vi "Test Get Sender from Nested Call Chain on Send.vi"(8 "error in (no error)":errorcluster, 11 "Test Case In":refnum<class "Debug Data Test.lvclass">) -> (0 "error out":errorcluster, 3 "Test Case Out":refnum<class "Debug Data Test.lvclass">)   [LabVIEW 2020, in "Debug Data Test.lvclass"]
uses:
  Debug Data Test.lvclass
  C:/Program Files (x86)/National Instruments/LabVIEW 2020/vi.lib/Astemes/LUnit/Test Case.lvclass
  source/Debug Data/Raw Debug Data.ctl
  source/Debug Data/Debug Data.lvclass/Debug Data.ctl
  <vilib>/Astemes/LUnit/Test Case.lvclass/Test Case.ctl
  <vilib>/Astemes/LUnit/LUnit Assertion Result.lvclass/LUnit Assertion Result.ctl
  <vilib>/Astemes/LUnit/LUnit Test Case Result.lvclass/LUnit Test Case Result.ctl
  <vilib>/Astemes/LUnit/LUnit Method Result.lvclass/LUnit Method Result.ctl
  01074fa8-ee8a-411d-bc8b-fc92c4f90959.vi
  <vilib>/Astemes/LUnit/Palette/Pass.vi
  <vilib>/Astemes/LUnit/Palette/Fail.vi
  <vilib>/Astemes/LUnit/Compare Variants.vi
  <vilib>/Astemes/LUnit/Describe Comparison.vi
  <vilib>/Astemes/LUnit/Set Assertion Type.vi
  <vilib>/Astemes/LUnit/Add test result.vi
  <vilib>/Astemes/LUnit/LUnit Write Passed.vi
  <vilib>/Astemes/LUnit/LUnit Write Message.vi
  <vilib>/Astemes/LUnit/LUnit Write Description.vi
  <vilib>/Astemes/LUnit/Variant to string.vi
  <vilib>/Astemes/LUnit/LUnit Write Assertion Type.vi
  <vilib>/Astemes/LUnit/LUnit Record Assertion Result.vi
  <vilib>/Astemes/LUnit/LUnit Aggregate Assertion Results.vi
  <vilib>/Astemes/LUnit/Assertion Result/LUnit Read Status.vi
  <vilib>/Astemes/LUnit/LUnit Read Message.vi
  <vilib>/Astemes/LUnit/LUnit Read Description.vi
  <vilib>/Astemes/LUnit/Method Result/LUnit Merge Status.vi
  <vilib>/Astemes/LUnit/LUnit Concatenate result strings.vi
  <vilib>/Utility/Data Type/Get Type Information.vi
  <vilib>/Utility/LVClass/Get LV Class Name.vi
  <vilib>/Astemes/LUnit/LUnit Assertion Result.lvclass
  Debug Data Test.lvclass/Debug Data Test.ctl
  source/Debug Data/Debug Data.lvclass
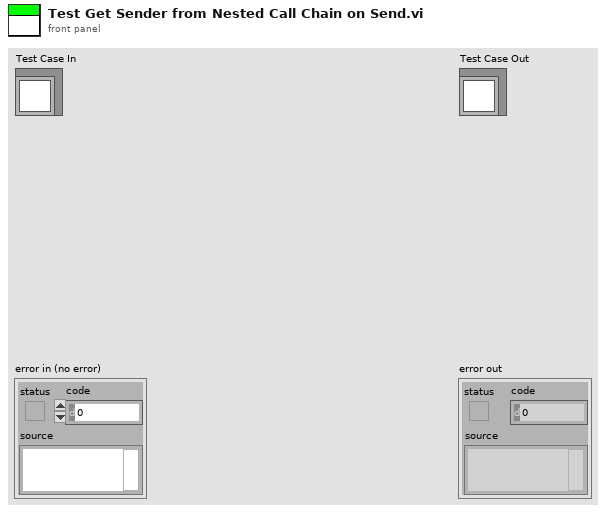
[diagram p1: front panel]
types:
  T1 = typedef "Debug Data.lvclass/Raw Debug Data.ctl" = cluster{"Action":string, "Call Chain":string, "Process":string, "Message":string, "Message Data":variant, "Time":dbl}
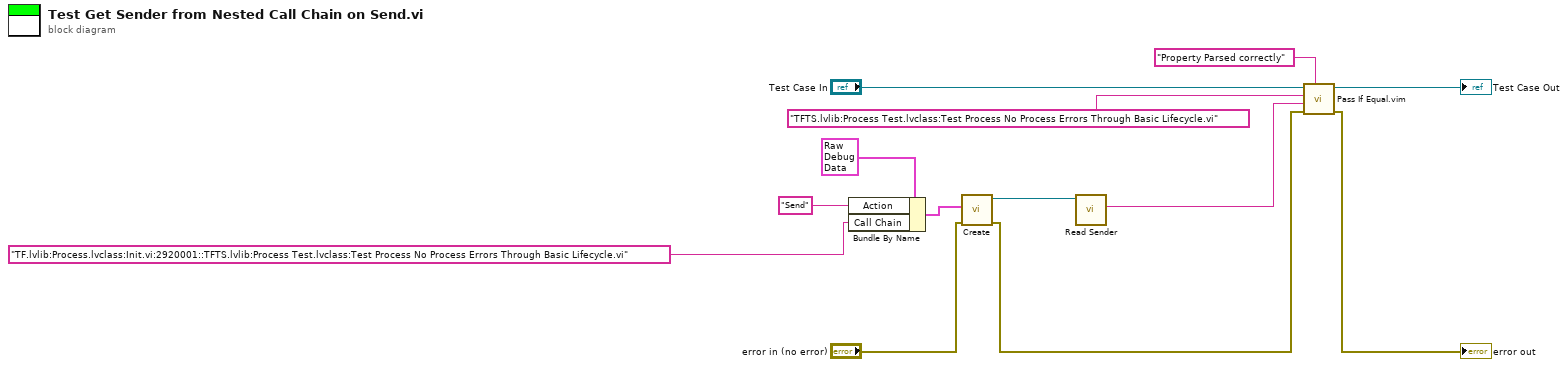
[diagram p0: block diagram]
diagram:
  n1 = Bundle By Name(cluster=T1 {"Action"="", "Call Chain"="", "Process"="", "Message"="", "Message Data"=variant, "Time"=0.0} ("Debug Data Cluster"), "Action"="Send", "Call Chain"="TF.lvlib:Process.lvclass:Init.vi:2920001::TFTS.lvlib:Process Test.lvclass:Test Process No Process Errors Through Basic Lifecycle.vi") -> (w9:T1)
  n2 = call "Create.vi"("error in (no error)"="error in (no error)", "Debug Data Cluster"=w9) -> ("error out"=w7:errorcluster, "Debug Data out"=w4:refnum<class "Debug Data.lvclass">)  [unwired: 8 in]
  n3 = call "Read Sender.vi"("Debug Data In"=w4) -> ("Sender"=w3:string)  [unwired: 9 in, 1 out]
  n4 = call "Pass If Equal.vim"("Description"="Property Parsed correctly", "error in (no error)"=w7, "Actual"=w3, "Expected"="TFTS.lvlib:Process Test.lvclass:Test Process No Process Errors Through Basic Lifecycle.vi", "LUnit Test Case In"="Test Case In") -> ("error out"=→"error out":errorcluster, "LUnit Test Case Out"=→"Test Case Out":refnum<class "Debug Data Test.lvclass">)  [unwired: 5 in]
